vi "ConvertAToGain.vi"(2 "String":string, 5 "error in":errorcluster) -> (16 "Gain":dbl, 19 "error out":errorcluster)   [LabVIEW 2018]
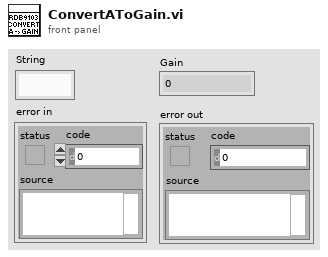
[diagram p1: front panel]
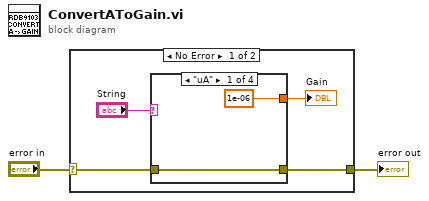
[diagram p0: block diagram]
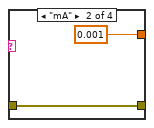
[diagram p2: hidden frame]
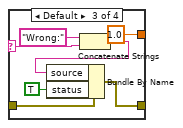
[diagram p3: hidden frame]
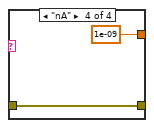
[diagram p4: hidden frame]
diagram:
  n1 = case shown="No Error" "error in" {
    selector: "error in" -> [w3 w20]
    tunnel: [w4 w20] -> w2
    frame No Error {
      n2 = case shown="\"uA\"" "String" {
        selector: "String" -> [_ _ w12 _]
        tunnel: [1e-06 ("Gain") 0.001 ("Gain") 1.0 ("Gain") 1e-09 ("Gain")] -> w5
        tunnel: w3 -> [w7 w9 w16 w18]
        tunnel: [w7 w9 w15 w18] -> w4
        frame "uA" {
        }
        frame "mA" {
        }
        frame Default {
          n3 = Concatenate Strings("Wrong:" ("source"), w12) -> (w11:string)
          n4 = Bundle By Name(cluster=w16, "source"=w11, "status"=TRUE) -> (w15:errorcluster)
        }
        frame "nA" {
        }
      }
      "Gain" <- w5
    }
    frame Error {
    }
  }
  "error out" <- w2
